vi "波形存储(子VI).vi"(9 "波形时间":timestamp, 10 "condition":string="ORP滴定曲线", 11 "ORP滴定曲线":u16[](graph)) -> ()   [LabVIEW 2016, in "斯坦道CODMn.lvlib"]
uses:
  <vilib>/Utility/sysdir.llb/System Directory Type.ctl
  <vilib>/Waveform/WDTFileIO.llb/ Write Waveform to File.vi
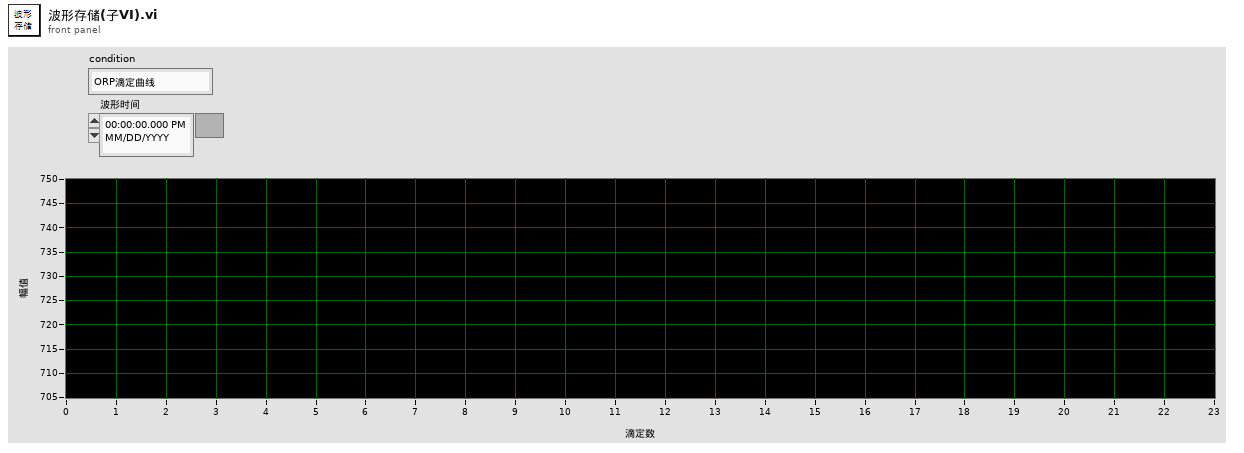
[diagram p1: front panel]
types:
  T1 = typedef "System Directory Type.ctl" = i32
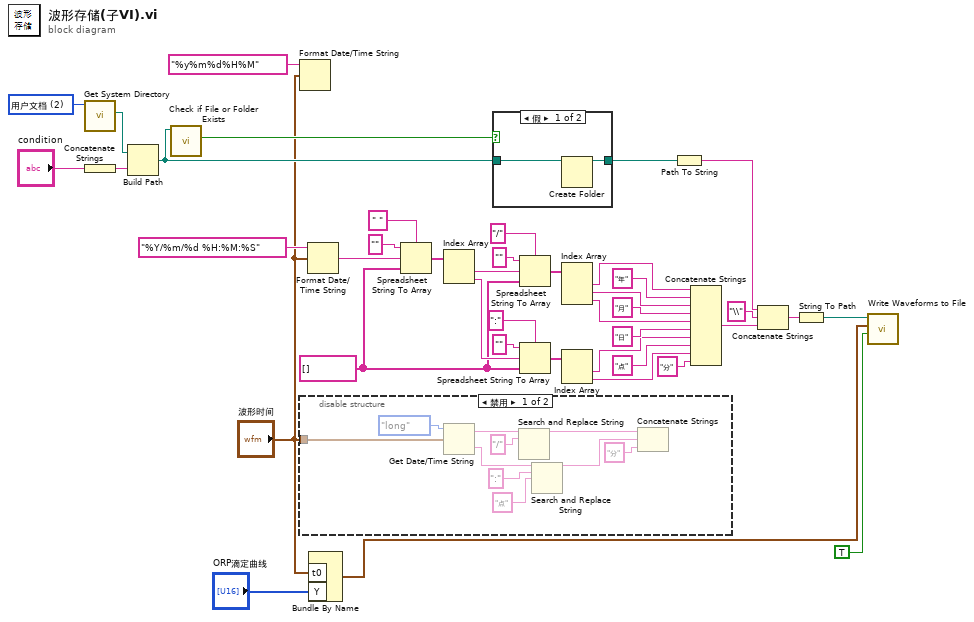
[diagram p0: block diagram]
diagram:
  w8 = string[] []
  w30 = T1 2 items=["用户目录"=0, "用户桌面"=1, "用户文档"=2, "用户应用程序数据"=3, "用户设置"=4, "用户临时目录"=5, "公共文档"=6, "公共应用程序数据"=7, "公共设置"=8, "公共缓存"=13, "系统核心库"=9, "系统安装库"=10, "应用程序文件"=11, "启动盘根目录"=12] ("system directory type")
  n1 = call <vilib>:"Get System Directory.vi"("system directory type"=w30) -> ("system directory"=w29:path)  [unwired: 10 in]
  n2 = Concatenate Strings("condition") -> (w27:string)
  n3 = Build Path(base path=w29, name or relative path=w27) -> (appended path=w32:path)
  n4 = call <vilib>:"Check if File or Folder Exists.vi"("path"=w32) -> ("file or folder exists?"=w31:bool)  [unwired: 8 in, 2 out]
  n5 = Format Date/Time String(time format string (%c)="%y%m%d%H%M" ("时间格式字符串(%c)"), seconds (now)="波形时间") -> ()  [unwired: 1 in, 1 out]
  n6 = disable-structure shown="禁用" {
    disable-tunnel: "波形时间" -> [w42 _]
    frame Disabled {
      n7 = Get Date/Time String(date format (0)=enum16{"short", "long", "abbreviated"}."long" ("日期格式(0)"), seconds (now)=w42) -> (date string=w45:string, time string=w47:string)  [unwired: 1 in]
      n8 = Search and Replace String(input string=w45, search string="/" ("搜索字符串")) -> (result string=w44:string)  [unwired: 6 in, 3 out]
      n9 = Search and Replace String(input string=w47, search string=":" ("搜索字符串"), replace string="点" ("替换字符串(\"\")")) -> (result string=w49:string)  [unwired: 5 in, 3 out]
      n10 = Concatenate Strings(w44, w49, "分" ("字符串")) -> ()  [unwired: 1 out]
    }
    frame Enabled {
    }
  }
  n11 = Format Date/Time String(time format string (%c)="%Y/%m/%d %H:%M:%S" ("时间格式字符串(%c)"), seconds (now)="波形时间") -> (date/time string=w2:string)  [unwired: 1 in]
  n12 = Bundle By Name("t0"="波形时间", "Y"="ORP滴定曲线") -> (w33:waveform(u16))  [unwired: 1 in]
  n13 = Spreadsheet String To Array(delimiter (Tab)=" " ("分隔符(Tab)"), format string="" ("格式字符串"), spreadsheet string=w2, array type (2D Dbl)=w8) -> (array=w23:string[])
  n14 = Index Array(array=w23) -> (element #1=w19:string, element #2=w9:string)  [unwired: 2 in]
  n15 = case shown="假" w31 {
    tunnel: w32 -> [w53 w54]
    tunnel: [w52 w54] -> w40
    frame False {
      n16 = Create Folder(path (use dialog)=w53) -> (created path=w52:path)  [unwired: 2 in, 2 out]
    }
    frame True {
    }
  }
  n17 = Spreadsheet String To Array(delimiter (Tab)="/" ("分隔符(Tab)"), format string="" ("格式字符串"), spreadsheet string=w19, array type (2D Dbl)=w8) -> (array=w18:string[])
  n18 = Spreadsheet String To Array(delimiter (Tab)=":" ("分隔符(Tab)"), format string="" ("格式字符串"), spreadsheet string=w9, array type (2D Dbl)=w8) -> (array=w7:string[])
  n19 = Index Array(array=w18) -> (element #1=w17:string, element #2=w15:string, element #3=w13:string)  [unwired: 3 in]
  n20 = Index Array(array=w7) -> (element #1=w6:string, element #2=w4:string)  [unwired: 2 in]
  n21 = Path To String(path=w40) -> (string=w34:string)
  n22 = Concatenate Strings(w17, "年" ("替换字符串(\"\")"), w15, "月" ("替换字符串(\"\")"), w13, "日" ("替换字符串(\"\")"), w6, "点" ("替换字符串(\"\")"), w4, "分" ("字符串")) -> (w1:string)
  n23 = Concatenate Strings(w34, "\\" ("字符串"), w1) -> (w36:string)
  n24 = String To Path(string=w36) -> (path=w37:path)
  n25 = call-poly <vilib>:"Write Waveforms to File.vi"("append to file? (new file:F)"=TRUE, "waveform"=w33, "file path (dialog if empty)"=w37) -> ()  [unwired: 7 in, 2 out]
